vi "LogHeaders.vi"(8 "error in":errorcluster, 10 "Date and Time":string, 11 "refnum in":refnum<file>) -> (0 "error out":errorcluster, 3 "refnum out":refnum<file>)   [LabVIEW 2018]
uses:
  DataNames.ctl
  LogOperation.ctl
  <vilib>/Rock Robotics/Network Tables/NT Read Number.vi
  <vilib>/Rock Robotics/Network Tables/NT Read String.vi
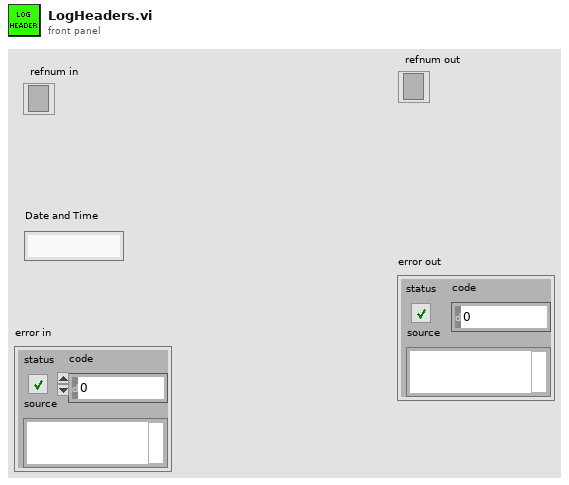
[diagram p1: front panel]
types:
  T1 = typedef "LogOperation.ctl" = enum16{"Set", "Get All", "Get Headers"}
  T2 = typedef "DataNames.ctl" = enum16{"RobotMode", "FMSConnected", "DriveLeft", "DriveRight", "EncoderLeft", "EncoderRight", "Angle", "LocationX", "LocationY", "CPU", "DriveOperation", "Battery"}
  T3 = typedef "NetComm_MatchType.ctl" = enum32{"None", "Practice", "Qualification", "Elimination"}
  T4 = typedef "WPI_DriverStationPositionInfo.ctl" = enum16{"1", "2", "3"}
  T5 = typedef "WPI_DriverStationAllianceInfo.ctl" = enum16{"Red", "Blue", "Invalid"}
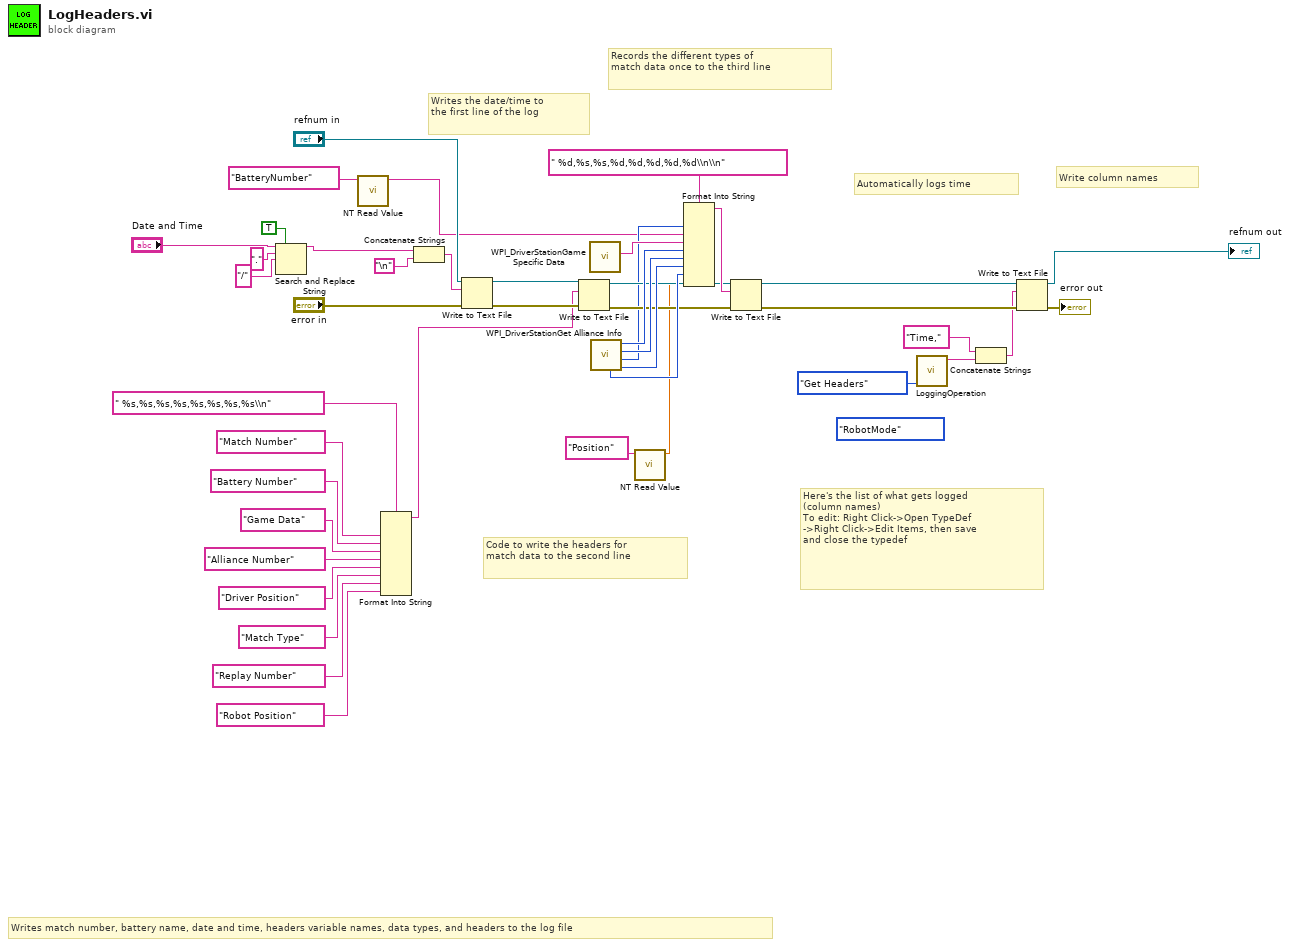
[diagram p0: block diagram]
diagram:
  (unwired) DataNames."RobotMode" ("Name")
  # "Here's the list of what gets logged\n(column names) \nTo edit: Right Click->Open TypeDef\n->Right Click->Edit Items, then save\nand close the typedef"
  # "Automatically logs time"
  # "Write column names"
  # "Records the different types of \nmatch data once to the third line"
  # "Code to write the headers for \nmatch data to the second line"
  # "Writes the date/time to\nthe first line of the log"
  # "Writes match number, battery name, date and time, headers variable names, data types, and headers to the log file"
  n1 = Search and Replace String(replace all?=TRUE ("replace all? (F)"), input string="Date and Time", search string=".", replace string="/" ("search string")) -> (result string=w11:string)  [unwired: 4 in, 3 out]
  n2 = call-poly <vilib>:"NT Read Value.vi"("Name"="BatteryNumber") -> ("String"=w5:string)  [unwired: 9 in, 1 out]
  n3 = Format Into String(format string=" %s,%s,%s,%s,%s,%s,%s,%s\\n", "Match Number" ("input 2"), "Battery Number" ("input 2"), "Game Data" ("input 2"), "Alliance Number" ("input 2"), "Driver Position" ("input 2"), "Match Type" ("input 2"), "Replay Number" ("input 2"), "Robot Position" ("input 2")) -> (resulting string=w16:string)  [unwired: 2 in, 1 out]
  n4 = Concatenate Strings(w11, "\n") -> (w42:string)
  n5 = Write to Text File(file (use dialog)="refnum in", text=w42, error in="error in") -> (refnum out=w28:refnum<file>, error out=w27:errorcluster)  [unwired: 1 in, 1 out]
  n6 = Write to Text File(file (use dialog)=w28, text=w16, error in=w27) -> (refnum out=w25:refnum<file>, error out=w26:errorcluster)  [unwired: 1 in, 1 out]
  n7 = call <vilib>:"WPI_DriverStationGame Specific Data.vi"() -> ("Game Specific Data"=w33:string)  [unwired: 11 in]
  n8 = call <vilib>:"WPI_DriverStationGet Alliance Info.vi"() -> ("Match Type"=w30:T3, "Match Number"=w7:u16, "Position"=w31:T4, "Alliance"=w32:T5, "Replay Number"=w29:u16)  [unwired: 6 in, 1 out]
  n9 = call-poly <vilib>:"NT Read Value.vi"("Name"="Position") -> ("Numeric"=w8:dbl)  [unwired: 9 in, 1 out]
  n10 = Format Into String(format string=" %d,%s,%s,%d,%d,%d,%d,%d\\n\\n", w7, w5, w33, w32, w31, w30, w29, w8) -> (resulting string=w39:string)  [unwired: 2 in, 1 out]
  n11 = Write to Text File(file (use dialog)=w25, text=w39, error in=w26) -> (refnum out=w38:refnum<file>, error out=w37:errorcluster)  [unwired: 1 in, 1 out]
  n12 = call "LoggingOperation.vi"("Operation"=LogOperation."Get Headers") -> ("Log String"=w2:string)  [unwired: 10 in]
  n13 = Concatenate Strings("Time," ("Column Name"), w2) -> (w3:string)
  n14 = Write to Text File(file (use dialog)=w38, text=w3, error in=w37) -> (refnum out=→"refnum out":refnum<file>, error out=→"error out":errorcluster)  [unwired: 1 in, 1 out]
